vi "GT_SetTrapPrm.vi"(3 "TrapPrm":T1, 4 "Profile in":T2=1 items=["Axis Control"=0, "Axis 1"=1, "Axis 2"=2, "Axis 3"=3, "Axis 4"=4, "Axis 5"=5, "Axis 6"=6, "Axis 7"=7, "Axis 8"=8, "Vector Space Control"=16, "Vector Space 1"=17, "Vector Space 2"=18, "Vector Space 3"=19, "Vector Space 4"=20], 5 "rtn_In":cluster{"rtn":i16, "Func":string}) -> (1 "Profile out":T2=1 items=["Axis Control"=0, "Axis 1"=1, "Axis 2"=2, "Axis 3"=3, "Axis 4"=4, "Axis 5"=5, "Axis 6"=6, "Axis 7"=7, "Axis 8"=8, "Vector Space Control"=16, "Vector Space 1"=17, "Vector Space 2"=18, "Vector Space 3"=19, "Vector Space 4"=20], 2 "rtn_Out":cluster{"rtn":i16, "Func":string})   [LabVIEW 2014]
uses:
  <vilib>/Motion/FlexMotion/CustomControls/CustomControls.llb/AxisOrVectorSpaceControl To Control.flx
  VC6/gts.dll
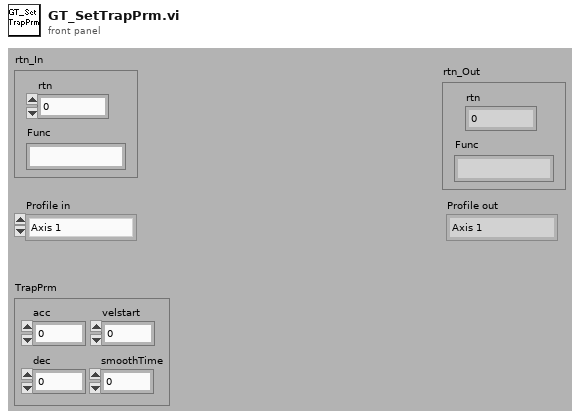
[diagram p1: front panel]
types:
  T1 = cluster{"acc":dbl, "dec":dbl, "velstart":dbl, "smoothTime":dbl}
  T2 = typedef "AxisOrVectorSpaceControl To Control.flx" = u16
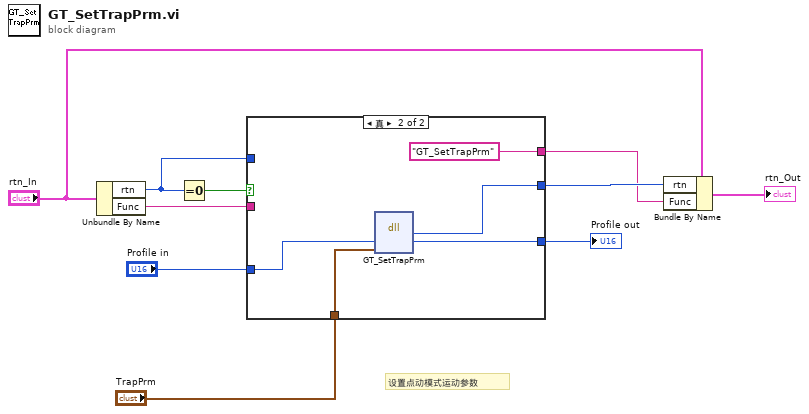
[diagram p0: block diagram]
diagram:
  # "设置点动模式运动参数"
  n1 = Unbundle By Name("rtn_In") -> ("rtn"=w3:i16, "Func"=w2:string)
  n2 = Equal To 0?(x=w3) -> (x = 0?=w10:bool)
  n3 = case shown="真" w10 {
    tunnel: "Profile in" -> [w13 w18]
    tunnel: [w13 w17] -> w8
    tunnel: [w12 w16] -> w6
    tunnel: [w11 "GT_SetTrapPrm" ("Func")] -> w5
    tunnel: w3 -> [w12 _]
    tunnel: w2 -> [w11 _]
    tunnel: "TrapPrm" -> [_ w14]
    frame False {
    }
    frame True {
      n4 = dll-call lib="PTH2Fabs DNewGTS AC-800LWin7版源程序-20170926gts85VC6gts.dll" fn="GT_SetTrapPrm"("profile"=w18, "TTrapPrm"=w14) -> ("rtn"=w16:i16, "profile"=w17:i16)  [unwired: 4 in, 2 out]
    }
  }
  "Profile out" <- w8
  n5 = Bundle By Name(cluster="rtn_In", "rtn"=w6, "Func"=w5) -> (→"rtn_Out":cluster{"rtn":i16, "Func":string})
